vi "Prognosis.vi"(5 "Day of Year":u32, 6 "Unique Object Identifier":string, 7 "Day Time":u32, 8 "Error In":errorcluster, 11 "DataFlowIN":T1) -> (0 "Error Out":errorcluster, 3 "DataFlowOUT":T1)   [LabVIEW 2017]
uses:
  classes/DataCollector.lvclass
  classes/DataHandler.lvclass
  classes/SimulationParameter.lvclass
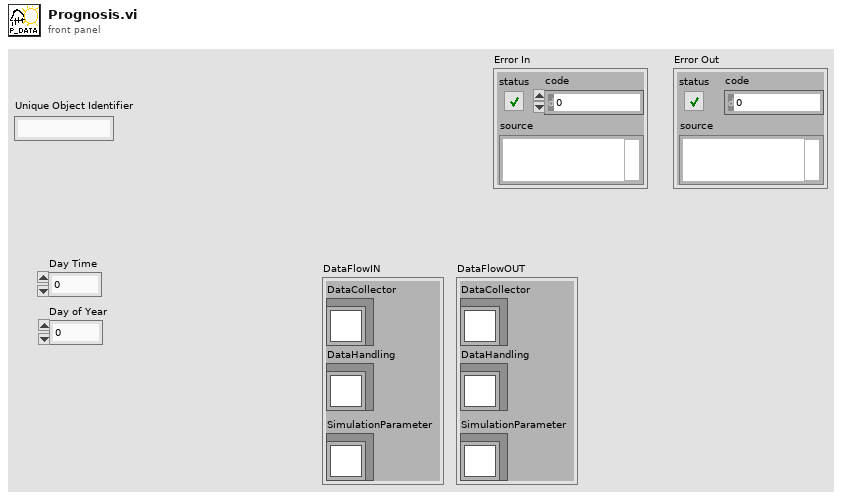
[diagram p1: front panel]
types:
  T1 = cluster{"DataCollector":refnum<class "DataCollector.lvclass">, "DataHandling":refnum<class "DataHandler.lvclass">, "SimulationParameter":refnum<class "SimulationParameter.lvclass">}
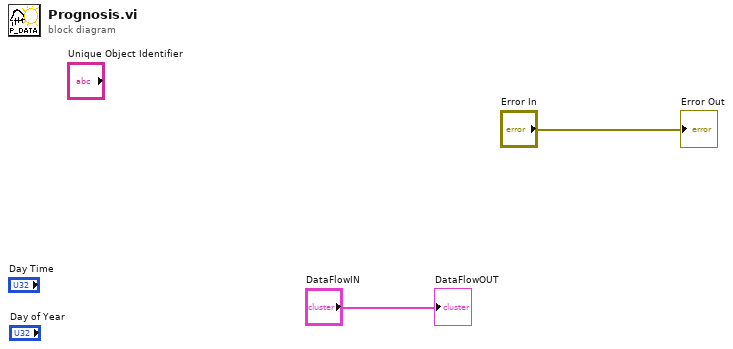
[diagram p0: block diagram]
diagram:
  "Error Out" <- "Error In"
  "DataFlowOUT" <- "DataFlowIN"
